vi "To OCU.vi"   [LabVIEW 2010]
uses:
  5.0-Global.vi
  4-High Neurons/Current GPS Data.ctl
  3-Midbrain/3.2-Where/_typedefs/3.2.1-VectorNav Data.ctl
  4-High Neurons/4.2-Where Sensor Typedef.ctl
  3-Midbrain/3.3-What/_typedefs/3.3.1-LIDAR Data Typedef.ctl
  4-High Neurons/4.3-What Sensor Typedef.ctl
  6-OCU Neurons/MainIndicators.ctl
  6-OCU Neurons/6.4-How Reporting Typedef.ctl
types:
  T1 = typedef "MainIndicators.ctl" = cluster{"Where?":bool, "What?":bool, "4.2-Where Am I? Sensor":T2, "4.3-What's Around Me? Sensor":T5, "5.3.1 MissionTimeAuto":dbl, "5.4 Clean How Am I? Sensor":T7, "How?":bool}
  T2 = typedef "4.2-Where Sensor Typedef.ctl" = cluster{"4.2.2- Current GPS Data":T3, "4.2.1-VectorNav Data":T4, "4.2.1-VectorNav Status":string}
  T3 = typedef "Current GPS Data.ctl" = cluster{"Lattitude (Decimal Degrees)":ext, "Longitude (Decimal Degrees)":ext, "EST Time":timestamp}
  T4 = typedef "3.2.1-VectorNav Data.ctl" = cluster{"Yaw":dbl, "Pitch":dbl, "Roll":dbl}
  T5 = typedef "4.3-What Sensor Typedef.ctl" = cluster{"LIDAR Data":T6}
  T6 = typedef "3.3.1-LIDAR Data Typedef.ctl" = cluster{"Angle array":dbl[], "Magnitude array ":dbl[]}
  T7 = typedef "6.4-How Reporting Typedef.ctl" = cluster{"Drive Speed (m/s)":dbl, "Lidar Inclination (deg) ":dbl, "Steering Angle (deg)":dbl, "Battery Voltage":dbl, "Drive Encoder Cable Check":bool, "Lidar Drive Encoder Cable Check":bool, "Steer Encoder Cable Check":bool, "Lidar Pos Encoder Cable Check":bool, "Mod Buttons & Blinky Cable Check":bool, "Lidar Data Cable Check":bool, "Drive Motor Cable Check":bool, "Vector Nav Cable Check":bool, "Lidar Drive Cable Check":bool, "Steer Drive Cable Check":bool, "Reverse?":bool, "Steering Control Voltage":dbl, "Drive Control Voltage":dbl, "Lidar Control Voltage":dbl}
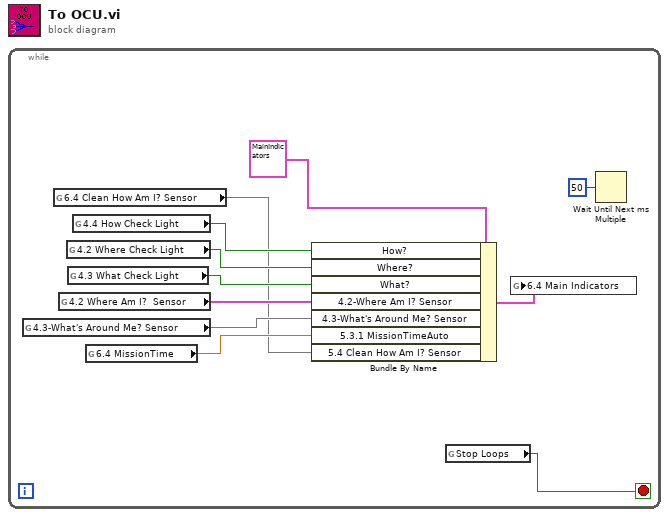
[diagram p0: block diagram]
diagram:
  n1 = while {
    stop <- w2 stop-if-true
    n2 = global read "5.0-Global.vi" "4.3-What's Around Me? Sensor"() -> (w7)
    n3 = global read "5.0-Global.vi" "6.4 Clean How Am I? Sensor"() -> (w3)
    n4 = global read "5.0-Global.vi" "4.2 Where Am I?  Sensor"() -> (w9:T2)
    n5 = global read "5.0-Global.vi" "4.2 Where Check Light"() -> (w5:bool)
    n6 = global read "5.0-Global.vi" "4.3 What Check Light"() -> (w8:bool)
    n7 = global read "5.0-Global.vi" "4.4 How Check Light"() -> (w6:bool)
    n8 = global read "5.0-Global.vi" "6.4 MissionTime"() -> (w4:dbl)
    n9 = Bundle By Name(cluster=T1 {"Where?"=FALSE, "What?"=FALSE, "4.2-Where Am I? Sensor"={"4.2.2- Current GPS Data"={"Lattitude (Decimal Degrees)"=0.0, "Longitude (Decimal Degrees)"=0.0, "EST Time"=timestamp(0 s since 1904-01-01)}, "4.2.1-VectorNav Data"={"Yaw"=0.0, "Pitch"=0.0, "Roll"=0.0}, "4.2.1-VectorNav Status"=""}, "4.3-What's Around Me? Sensor"={"LIDAR Data"={"Angle array"=[], "Magnitude array "=[]}}, "5.3.1 MissionTimeAuto"=0.0, "5.4 Clean How Am I? Sensor"={"Drive Speed (m/s)"=0.0, "Lidar Inclination (deg) "=0.0, "Steering Angle (deg)"=0.0, "Battery Voltage"=0.0, "Drive Encoder Cable Check"=FALSE, "Lidar Drive Encoder Cable Check"=FALSE, "Steer Encoder Cable Check"=FALSE, "Lidar Pos Encoder Cable Check"=FALSE, "Mod Buttons & Blinky Cable Check"=FALSE, "Lidar Data Cable Check"=FALSE, "Drive Motor Cable Check"=FALSE, "Vector Nav Cable Check"=FALSE, "Lidar Drive Cable Check"=FALSE, "Steer Drive Cable Check"=FALSE, "Reverse?"=FALSE, "Steering Control Voltage"=0.0, "Drive Control Voltage"=0.0, "Lidar Control Voltage"=0.0}, "How?"=FALSE} ("5.7.2 Main Indicators"), "How?"=w6, "Where?"=w5, "What?"=w8, "4.2-Where Am I? Sensor"=w9, "4.3-What's Around Me? Sensor"=w7, "5.3.1 MissionTimeAuto"=w4, "5.4 Clean How Am I? Sensor"=w3) -> (w10:T1)
    n10 = global read "5.0-Global.vi" "Stop Loops"() -> (w2:bool)
    n11 = global write "5.0-Global.vi" "6.4 Main Indicators"(w10) -> ()
    n12 = Wait Until Next ms Multiple(millisecond multiple=u32 50) -> ()  [unwired: 1 out]
  }
